vi "global variable.vi"() -> ()   [LabVIEW 2020]
uses:
  composed-event-logger/Source/ConsoleView/ConsoleInterface/ConsoleSession.lvclass
panel:
  in  "ConsoleSession out":refnum<class "ConsoleSession.lvclass">
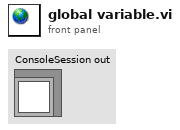
[diagram p1: front panel]
diagram:
